vi "ASI_change_Z_speed.vi"(2 "error in (no error)":errorcluster, 3 "VISA resource name":refnum<visa-resource-name>="COM7", 4 "speed":dbl) -> (0 "error out":errorcluster, 1 "VISA resource name out":refnum<visa-resource-name>)   [LabVIEW 2015]
uses:
  <vilib>/Instr/_visa.llb/VISA Flush IO Buffer Mask.ctl
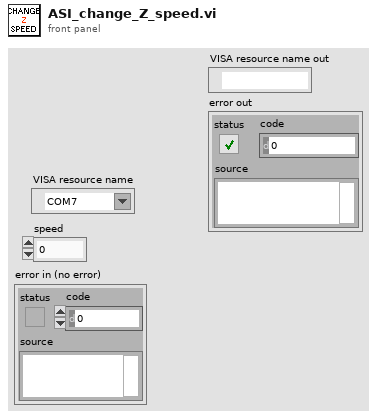
[diagram p1: front panel]
types:
  T1 = typedef "VISA Flush IO Buffer Mask.ctl" = u16
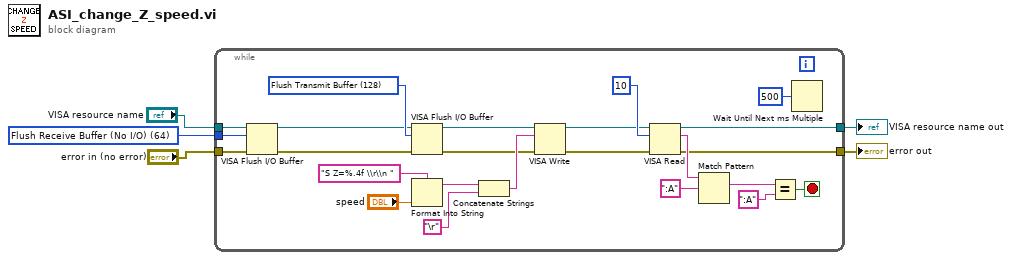
[diagram p0: block diagram]
diagram:
  w4 = T1 64 items=["Flush Receive Buffer"=16, "Write Transmit Buffer to Device"=32, "Flush Receive Buffer (No I/O)"=64, "Flush Transmit Buffer"=128] ("Mask")
  n1 = while {
    tunnel: "error in (no error)" -> [w27]
    tunnel: w4 -> [w21]
    tunnel: "VISA resource name" -> [w20]
    tunnel: [w7] -> w1
    tunnel: [w8] -> w2
    stop <- w12 stop-if-true
    w24 = T1 128 items=["Flush Receive Buffer"=16, "Write Transmit Buffer to Device"=32, "Flush Receive Buffer (No I/O)"=64, "Flush Transmit Buffer"=128] ("Mask")
    n2 = VISA Flush I/O Buffer(VISA resource name=w20, mask (16)=w21, error in (no error)=w27) -> (VISA resource name out=w23:refnum<visa-resource-name>, error out=w22:errorcluster)
    n3 = VISA Flush I/O Buffer(VISA resource name=w23, mask (16)=w24, error in (no error)=w22) -> (VISA resource name out=w26:refnum<visa-resource-name>, error out=w25:errorcluster)
    n4 = Format Into String(format string="S Z=%.4f \\r\\n ", "speed") -> (resulting string=w6:string)  [unwired: 2 in, 1 out]
    n5 = Concatenate Strings(w6, "\r") -> (w28:string)
    n6 = VISA Write(VISA resource name=w26, write buffer=w28, error in (no error)=w25) -> (VISA resource name out=w10:refnum<visa-resource-name>, error out=w13:errorcluster)  [unwired: 1 out]
    n7 = VISA Read(VISA resource name=w10, byte count=u32 10, error in (no error)=w13) -> (VISA resource name out=w8:refnum<visa-resource-name>, read buffer=w16:string, error out=w7:errorcluster)  [unwired: 1 out]
    n8 = Match Pattern(string=w16, regular expression=":A" ("y")) -> (match substring=w17:string)  [unwired: 1 in, 3 out]
    n9 = Equal?(x=w17, y=":A") -> (x = y?=w12:bool)
    n10 = Wait Until Next ms Multiple(millisecond multiple=u32 500) -> ()  [unwired: 1 out]
  }
  "VISA resource name out" <- w2
  "error out" <- w1
